vi "Get Host IP Address.vi"(8 "error in (no error)":errorcluster) -> (0 "error out":errorcluster, 3 "Host IP Address":string)   [LabVIEW 2016, in "Assert API Components.lvlib" / "Log Assert Core.lvlib"]
uses:
  Log Assert Core.lvlib
  <vilib>/Utility/config.llb/Read Key (String).vi
  <vilib>/Utility/config.llb/NI_LVConfig.lvlib
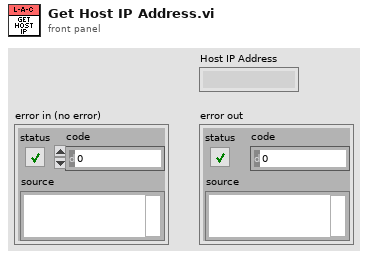
[diagram p1: front panel]
types:
  T1 = typedef "NI_LVConfig.lvlib/Config Data RefNum.ctl" = refnum<k1>
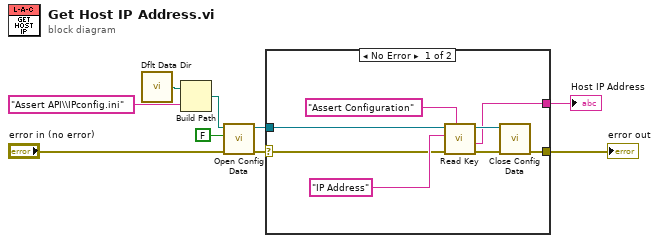
[diagram p0: block diagram]
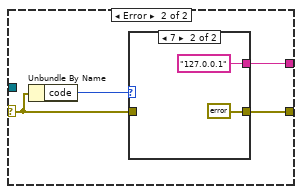
[diagram p2: hidden frame]
diagram:
  n1 = call <vilib>:"Dflt Data Dir.vi"() -> ("App:Default Data Directory"=w2:path)
  n2 = Build Path(base path=w2, name or relative path="Assert API\\IPconfig.ini") -> (appended path=w4:path)
  n3 = call <vilib>:"Open Config Data.vi"("error in (no error)"="error in (no error)", "create file if necessary (T)"=FALSE, "configuration file path"=w4) -> ("error out"=w6:errorcluster, "refnum"=w7:T1)  [unwired: 6 in, 1 out]
  n4 = case shown="No Error" w6 {
    selector: w6 -> [w14 w19]
    tunnel: w7 -> [w15 _]
    tunnel: [w10 w20] -> w9
    tunnel: [w11 w18] -> w8
    frame No Error {
      n5 = call-poly <vilib>:"Read Key.vi"("section"="Assert Configuration", "error in (no error)"=w14, "key"="IP Address", "refnum"=w15) -> ("error out"=w12:errorcluster, "value"=w10:string, "refnum out"=w13:T1)  [unwired: 4 in, 1 out]
      n6 = call <vilib>:"Close Config Data.vi"("error in (no error)"=w12, "refnum"=w13) -> ("error out"=w11:errorcluster)  [unwired: 8 in, 1 out]
    }
    frame Error {
      n7 = Unbundle By Name(w19) -> ("code"=w21:i32)
      n8 = case shown="7" w21 {
        tunnel: [_ "127.0.0.1"] -> w20
        tunnel: w19 -> [w22 _]
        tunnel: [w22 errorcluster {"status"=FALSE, "code"=0, "source"=""} ("error IO")] -> w18
        frame Default {
        }
        frame 7 {
        }
      }
    }
  }
  "Host IP Address" <- w9
  "error out" <- w8
